vi "Script New Cases in Case Structure - Target VI.vi"() -> ()   [LabVIEW 2020]
panel:
  in  "Numeric":i32
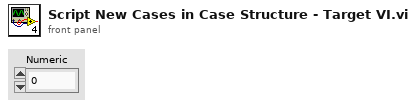
[diagram p1: front panel]
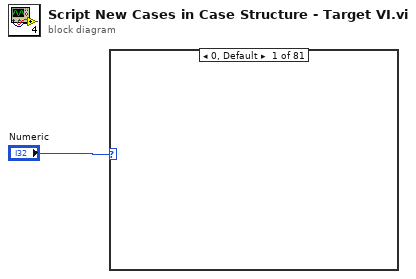
[diagram p0: block diagram]
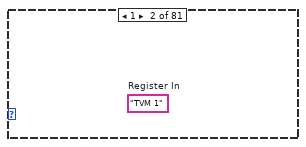
[diagram p2: hidden frame]
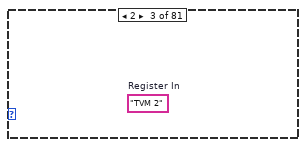
[diagram p3: hidden frame]
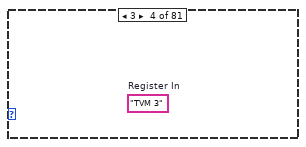
[diagram p4: hidden frame]
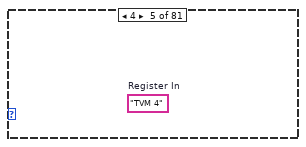
[diagram p5: hidden frame]
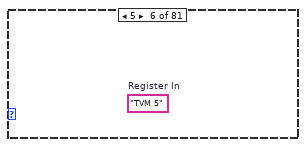
[diagram p6: hidden frame]
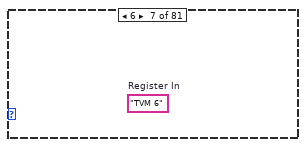
[diagram p7: hidden frame]
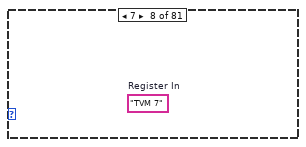
[diagram p8: hidden frame]
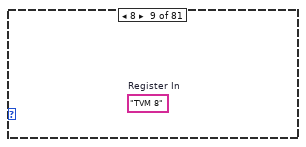
[diagram p9: hidden frame]
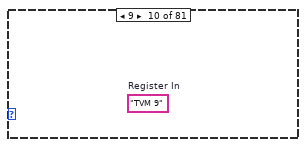
[diagram p10: hidden frame]
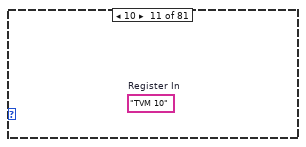
[diagram p11: hidden frame]
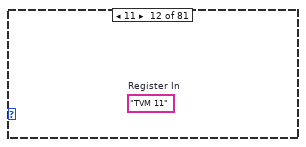
[diagram p12: hidden frame]
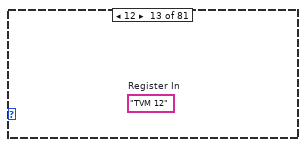
[diagram p13: hidden frame]
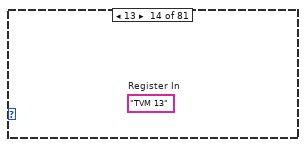
[diagram p14: hidden frame]
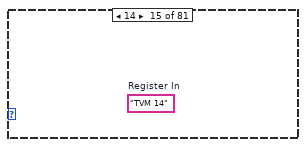
[diagram p15: hidden frame]
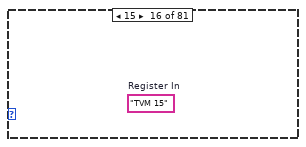
[diagram p16: hidden frame]
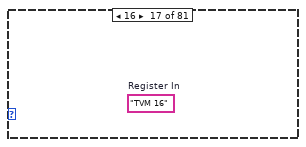
[diagram p17: hidden frame]
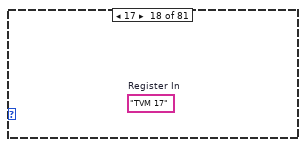
[diagram p18: hidden frame]
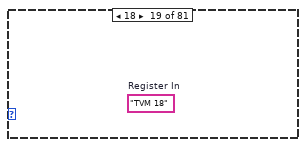
[diagram p19: hidden frame]
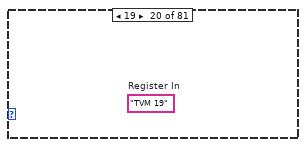
[diagram p20: hidden frame]
diagram:
  n1 = case shown="0, Default" "Numeric" {
    frame 0, Default {
    }
    frame 1 {
      (unwired) "TVM 1"  # Register In
    }
    frame 2 {
      (unwired) "TVM 2"  # Register In
    }
    frame 3 {
      (unwired) "TVM 3"  # Register In
    }
    frame 4 {
      (unwired) "TVM 4"  # Register In
    }
    frame 5 {
      (unwired) "TVM 5"  # Register In
    }
    frame 6 {
      (unwired) "TVM 6"  # Register In
    }
    frame 7 {
      (unwired) "TVM 7"  # Register In
    }
    frame 8 {
      (unwired) "TVM 8"  # Register In
    }
    frame 9 {
      (unwired) "TVM 9"  # Register In
    }
    frame 10 {
      (unwired) "TVM 10"  # Register In
    }
    frame 11 {
      (unwired) "TVM 11"  # Register In
    }
    frame 12 {
      (unwired) "TVM 12"  # Register In
    }
    frame 13 {
      (unwired) "TVM 13"  # Register In
    }
    frame 14 {
      (unwired) "TVM 14"  # Register In
    }
    frame 15 {
      (unwired) "TVM 15"  # Register In
    }
    frame 16 {
      (unwired) "TVM 16"  # Register In
    }
    frame 17 {
      (unwired) "TVM 17"  # Register In
    }
    frame 18 {
      (unwired) "TVM 18"  # Register In
    }
    frame 19 {
      (unwired) "TVM 19"  # Register In
    }
    frame 20 {
      (unwired) "TVM 20"  # Register In
    }
    frame 21 {
      (unwired) "TVM 21"  # Register In
    }
    frame 22 {
      (unwired) "TVM 22"  # Register In
    }
    frame 23 {
      (unwired) "TVM 23"  # Register In
    }
    frame 24 {
      (unwired) "TVM 24"  # Register In
    }
    frame 25 {
      (unwired) "TVM 25"  # Register In
    }
    frame 26 {
      (unwired) "TVM 26"  # Register In
    }
    frame 27 {
      (unwired) "TVM 27"  # Register In
    }
    frame 28 {
      (unwired) "TVM 28"  # Register In
    }
    frame 29 {
      (unwired) "TVM 29"  # Register In
    }
    frame 30 {
      (unwired) "TVM 30"  # Register In
    }
    frame 31 {
      (unwired) "TVM 31"  # Register In
    }
    frame 32 {
      (unwired) "TVM 32"  # Register In
    }
    frame 33 {
      (unwired) "TVM 33"  # Register In
    }
    frame 34 {
      (unwired) "TVM 34"  # Register In
    }
    frame 35 {
      (unwired) "TVM 35"  # Register In
    }
    frame 36 {
      (unwired) "TVM 36"  # Register In
    }
    frame 37 {
      (unwired) "TVM 37"  # Register In
    }
    frame 38 {
      (unwired) "TVM 38"  # Register In
    }
    frame 39 {
      (unwired) "TVM 39"  # Register In
    }
    frame 40 {
      (unwired) "TVM 40"  # Register In
    }
    frame 41 {
      (unwired) "TVM 41"  # Register In
    }
    frame 42 {
      (unwired) "TVM 42"  # Register In
    }
    frame 43 {
      (unwired) "TVM 43"  # Register In
    }
    frame 44 {
      (unwired) "TVM 44"  # Register In
    }
    frame 45 {
      (unwired) "TVM 45"  # Register In
    }
    frame 46 {
      (unwired) "TVM 46"  # Register In
    }
    frame 47 {
      (unwired) "TVM 47"  # Register In
    }
    frame 48 {
      (unwired) "TVM 48"  # Register In
    }
    frame 49 {
      (unwired) "TVM 49"  # Register In
    }
    frame 50 {
      (unwired) "TVM 50"  # Register In
    }
    frame 51 {
      (unwired) "TVM 51"  # Register In
    }
    frame 52 {
      (unwired) "TVM 52"  # Register In
    }
    frame 53 {
      (unwired) "TVM 53"  # Register In
    }
    frame 54 {
      (unwired) "TVM 54"  # Register In
    }
    frame 55 {
      (unwired) "TVM 55"  # Register In
    }
    frame 56 {
      (unwired) "TVM 56"  # Register In
    }
    frame 57 {
      (unwired) "TVM 57"  # Register In
    }
    frame 58 {
      (unwired) "TVM 58"  # Register In
    }
    frame 59 {
      (unwired) "TVM 59"  # Register In
    }
    frame 60 {
      (unwired) "TVM 60"  # Register In
    }
    frame 61 {
      (unwired) "TVM 61"  # Register In
    }
    frame 62 {
      (unwired) "TVM 62"  # Register In
    }
    frame 63 {
      (unwired) "TVM 63"  # Register In
    }
    frame 64 {
      (unwired) "TVM 64"  # Register In
    }
    frame 65 {
      (unwired) "TVM 65"  # Register In
    }
    frame 66 {
      (unwired) "TVM 66"  # Register In
    }
    frame 67 {
      (unwired) "TVM 67"  # Register In
    }
    frame 68 {
      (unwired) "TVM 68"  # Register In
    }
    frame 69 {
      (unwired) "TVM 69"  # Register In
    }
    frame 70 {
      (unwired) "TVM 70"  # Register In
    }
    frame 71 {
      (unwired) "TVM 71"  # Register In
    }
    frame 72 {
      (unwired) "TVM 72"  # Register In
    }
    frame 73 {
      (unwired) "TVM 73"  # Register In
    }
    frame 74 {
      (unwired) "TVM 74"  # Register In
    }
    frame 75 {
      (unwired) "TVM 75"  # Register In
    }
    frame 76 {
      (unwired) "TVM 76"  # Register In
    }
    frame 77 {
      (unwired) "TVM 77"  # Register In
    }
    frame 78 {
      (unwired) "TVM 78"  # Register In
    }
    frame 79 {
      (unwired) "TVM 79"  # Register In
    }
    frame 80 {
      (unwired) "TVM 80"  # Register In
    }
  }
